vi "Valve Type.vi"(11 "Valve in":refnum<class "ValveControl.lvclass">) -> (2 "Valve Type":string)   [LabVIEW 2020, in "VolatusControl.lvlib" / "ValveControl.lvclass"]
uses:
  ValveControl.lvclass
  ValveControl.lvclass/ValveControl.ctl
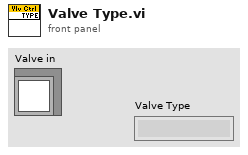
[diagram p1: front panel]
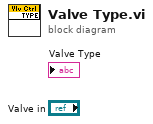
[diagram p0: block diagram]
diagram:
